vi "JSON to CANbus data.vi"(7 "Database Alias":string, 8 "error in":errorcluster, 11 "JSON file":path) -> (0 "error out":errorcluster, 3 "Signal Sessions":T1)   [LabVIEW 2021]
uses:
  controls/JSON sigs.ctl
  ceb00c8f-060c-42ee-8538-48eed6d5856c.vi
  <vilib>/JDP Science/JSONtext/JSON text to Variant.vi
  <vilib>/JDP Science/JSONtext/LVClass Serializer/JSONtext LVClass Serializer.lvclass
panel:
  out "JSON string":string
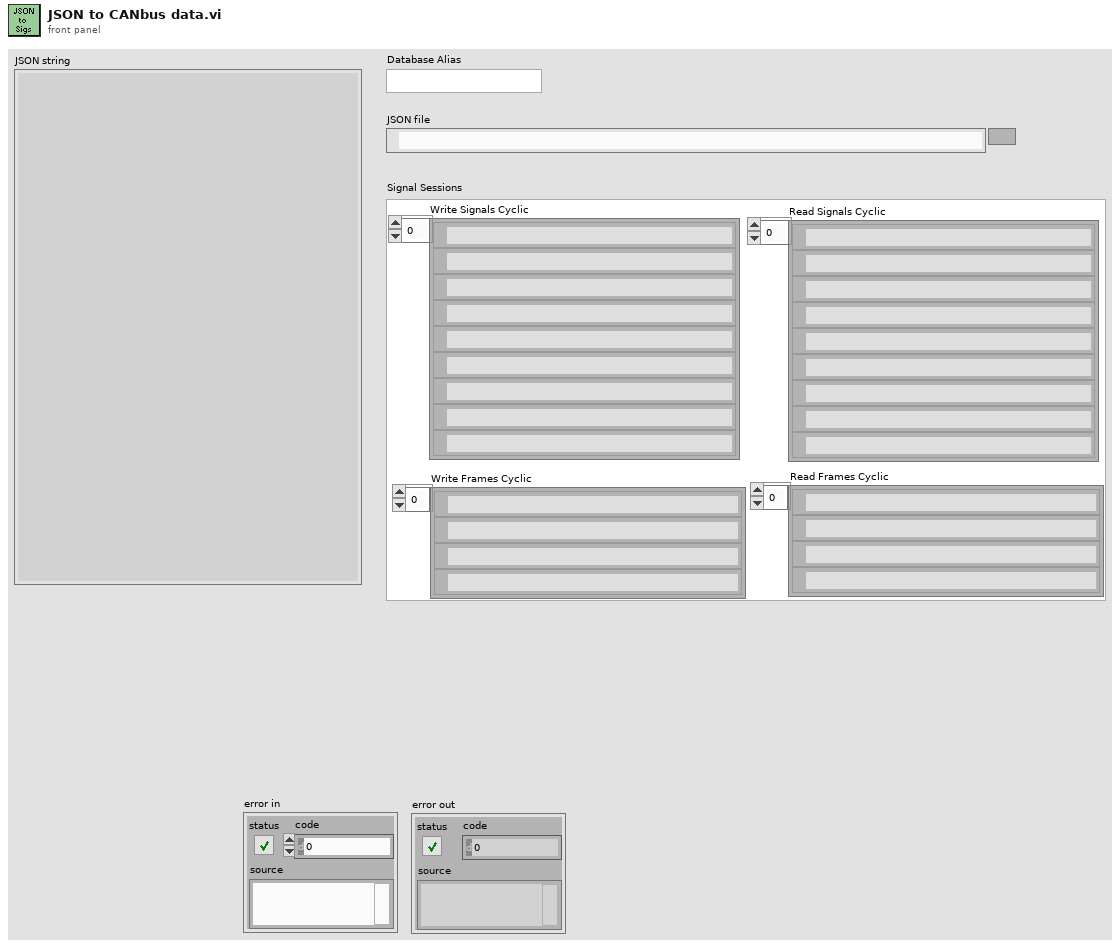
[diagram p1: front panel]
types:
  T1 = typedef "JSON sigs.ctl" = cluster{"Read Signals Cyclic":refnum<k21>[], "Write Signals Cyclic":refnum<k21>[], "Write Frames Cyclic":refnum<k21>[], "Read Frames Cyclic":refnum<k21>[]}
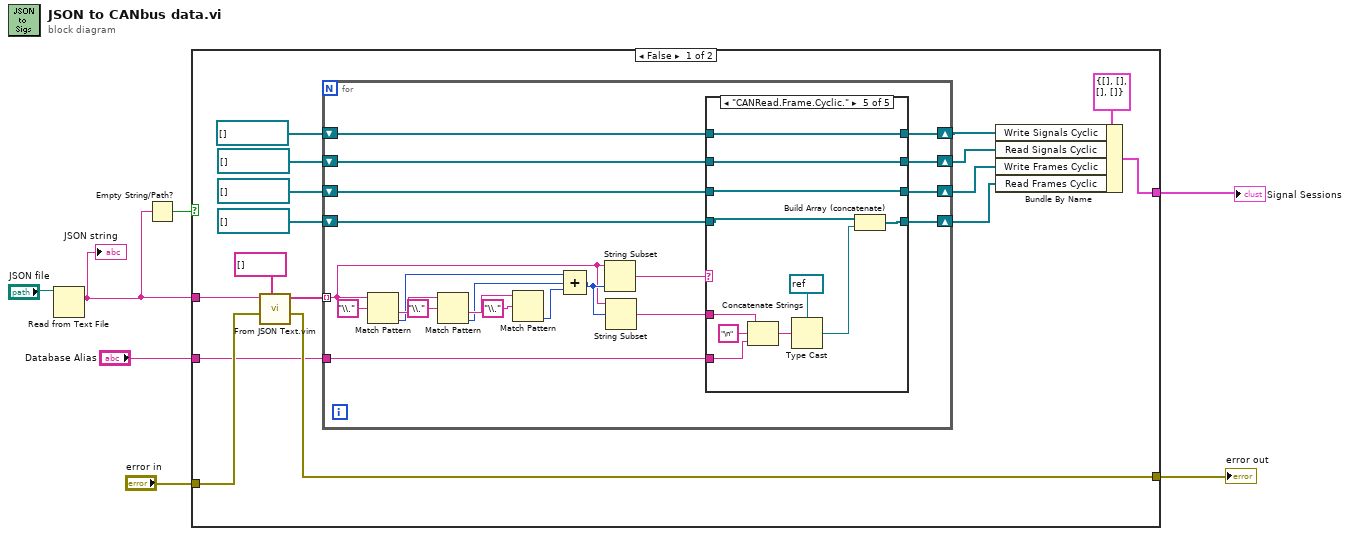
[diagram p0: block diagram]
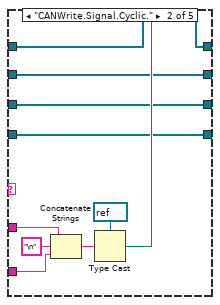
[diagram p3: hidden frame]
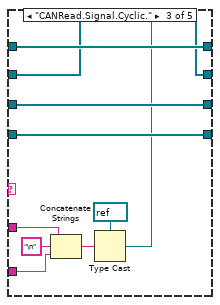
[diagram p4: hidden frame]
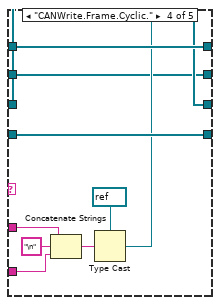
[diagram p5: hidden frame]
diagram:
  n1 = Read from Text File(file (use dialog)="JSON file") -> (text=w1:string)  [unwired: 3 in, 3 out]
  "JSON string" <- w1
  n2 = Empty String/Path?(string/path=w1) -> (empty?=w5:bool)
  n3 = case shown="False" w5 {
    tunnel: [w20 _] -> w7
    tunnel: "error in" -> [w11 w93]
    tunnel: w1 -> [w10 _]
    tunnel: [w9 w93] -> w4
    tunnel: "Database Alias" -> [w8 _]
    frame False {
      n4 = call "From JSON Text.vim"("Data Type and Default Value"=string[] [] ("regular expression"), "error in (no error)"=w11, "JSON"=w10) -> ("error out"=w9:errorcluster, "Data out"=w22:string[])  [unwired: 7 in]
      n5 = for {
        tunnel: w22 -> [w35] mode=indexing
        tunnel: w8 -> [w34]
        shift-right: [w29] -> w15
        shift-left: refnum<k21>[] [] ("Read Signals Cyclic") -> [w33]
        shift-right: [w28] -> w14
        shift-left: refnum<k21>[] [] ("Read Signals Cyclic") -> [w32]
        shift-right: [w27] -> w13
        shift-left: refnum<k21>[] [] ("Write Frames Cyclic") -> [w31]
        shift-right: [w26] -> w12
        shift-left: refnum<k21>[] [] ("Write Frames Cyclic") -> [w30]
        n6 = Match Pattern(string=w35, regular expression="\\.") -> (after substring=w41:string, offset past match=w39:i32)  [unwired: 1 in, 2 out]
        n7 = Match Pattern(string=w41, regular expression="\\.") -> (after substring=w40:string, offset past match=w38:i32)  [unwired: 1 in, 2 out]
        n8 = Match Pattern(string=w40, regular expression="\\.") -> (offset past match=w37:i32)  [unwired: 1 in, 3 out]
        n9 = Compound Arithmetic op=ADD(w39, w38, w37) -> (w36:i32)
        n10 = String Subset(string=w35, length (rest)=w36) -> (substring=w25:string)  [unwired: 1 in]
        n11 = String Subset(string=w35, offset (0)=w36) -> (substring=w24:string)  [unwired: 1 in]
        n12 = case shown="\"CANRead.Frame.Cyclic.\"" w25 {
          tunnel: w24 -> [_ w56 w67 w79 w90]
          tunnel: w34 -> [_ w55 w66 w78 w89]
          tunnel: w33 -> [w48 w53 w63 w76 w88]
          tunnel: w32 -> [w47 w51 w60 w73 w87]
          tunnel: w31 -> [w46 w50 w65 w72 w83]
          tunnel: w30 -> [w45 w49 w64 w77 w82]
          tunnel: [w48 w52 w63 w76 w88] -> w29
          tunnel: [w47 w51 w62 w73 w87] -> w28
          tunnel: [w46 w50 w65 w75 w83] -> w27
          tunnel: [w45 w49 w64 w77 w85] -> w26
          frame Default {
          }
          frame "CANWrite.Signal.Cyclic." {
            n13 = Concatenate Strings(w56, "\n" ("string"), w55) -> (w59:string)
            n14 = Type Cast(type=refnum<k21> refnum ("XNET Signal"), x=w59) -> (*(type *) &x=w54:refnum<k21>)
            n15 = Build Array (concatenate)(w53, w54) -> (w52:refnum<k21>[])
          }
          frame "CANRead.Signal.Cyclic." {
            n16 = Concatenate Strings(w67, "\n" ("string"), w66) -> (w70:string)
            n17 = Type Cast(type=refnum<k21> refnum ("XNET Signal"), x=w70) -> (*(type *) &x=w61:refnum<k21>)
            n18 = Build Array (concatenate)(w60, w61) -> (w62:refnum<k21>[])
          }
          frame "CANWrite.Frame.Cyclic." {
            n19 = Concatenate Strings(w79, "\n" ("string"), w78) -> (w81:string)
            n20 = Type Cast(type=refnum<k21> refnum ("Frame Name"), x=w81) -> (*(type *) &x=w74:refnum<k21>)
            n21 = Build Array (concatenate)(w72, w74) -> (w75:refnum<k21>[])
          }
          frame "CANRead.Frame.Cyclic." {
            n22 = Concatenate Strings(w90, "\n" ("string"), w89) -> (w92:string)
            n23 = Type Cast(type=refnum<k21> refnum ("Frame Name"), x=w92) -> (*(type *) &x=w84:refnum<k21>)
            n24 = Build Array (concatenate)(w82, w84) -> (w85:refnum<k21>[])
          }
        }
      }
      n25 = Bundle By Name(cluster=T1 {"Read Signals Cyclic"=[], "Write Signals Cyclic"=[], "Write Frames Cyclic"=[], "Read Frames Cyclic"=[]} ("Signal Sessions"), "Write Signals Cyclic"=w15, "Read Signals Cyclic"=w14, "Write Frames Cyclic"=w13, "Read Frames Cyclic"=w12) -> (w20:T1)
    }
    frame True {
    }
  }
  "Signal Sessions" <- w7
  "error out" <- w4
